vi "Cat action vi.vi"(1 "i":i32, 2 "Action":enum16{"Cat", "Jump", "Fall", "Fly", "Rote"}(ring)) -> (0 "Game Cat":u16(ring))   [LabVIEW 2010]
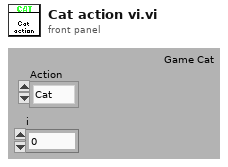
[diagram p1: front panel]
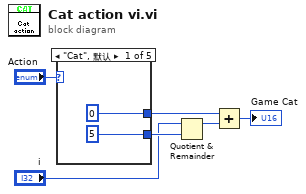
[diagram p0: block diagram]
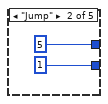
[diagram p2: hidden frame]
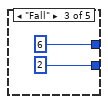
[diagram p3: hidden frame]
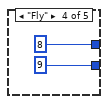
[diagram p4: hidden frame]
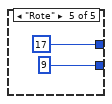
[diagram p5: hidden frame]
diagram:
  n1 = case shown="\"Cat\", 默认" "Action" {
    tunnel: [0 5 6 8 17] -> w4
    tunnel: [5 1 2 9 9] -> w3
    frame "Cat", Default {
    }
    frame "Jump" {
    }
    frame "Fall" {
    }
    frame "Fly" {
    }
    frame "Rote" {
    }
  }
  n2 = Quotient & Remainder(x="i", y=w3) -> (x-y*floor(x/y)=w6:i32)  [unwired: 1 out]
  n3 = Add(x=w4, y=w6) -> (x+y=→"Game Cat":i32)
